vi "Construct MCListbox Item Names Binding.vi"(9 "Set to top left upon write? (F)":T1, 10 "MCListbox Refnum":refnum<vi>) -> (0 "error out":errorcluster, 3 "MCListboxItemNamesBinding":refnum<class "MCListboxItemNamesBinding.lvclass">)   [LabVIEW 2017, in "MCListboxItemNamesBinding.lvclass"]
doc: "<License>\nCopyright © 2017 Composed Systems, LLC | All rights reserved\nwww.composed.io\n\nAuthor: Ethan Stern <ethan.stern@composed.io>\n\nThis software is provided \"AS IS\" WITHOUT WARRANTIES, either express or implied, AND IS FOR EDUCATIONAL PURPOSES ONLY.\n</License>"
uses:
  MCListboxItemNamesBinding.lvclass
  MCListbox Binding Options.ctl
  MCListboxItemNamesBinding.lvclass/MCListboxItemNamesBinding.ctl
  <vilib>/Utility/error.llb/Error Cluster From Error Code.vi
  <vilib>/ErrorRing/Error Ring.xnode
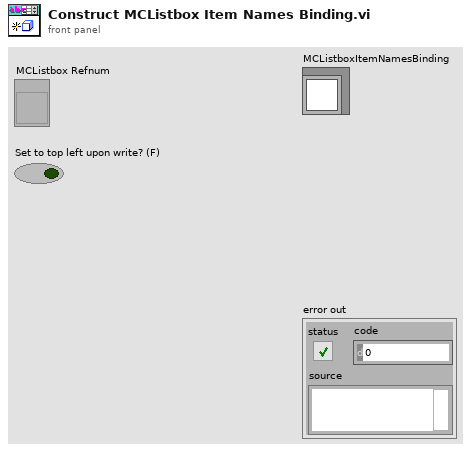
[diagram p1: front panel]
types:
  T1 = typedef "MCListboxItemNamesBinding.lvclass/MCListbox Binding Options.ctl" = bool
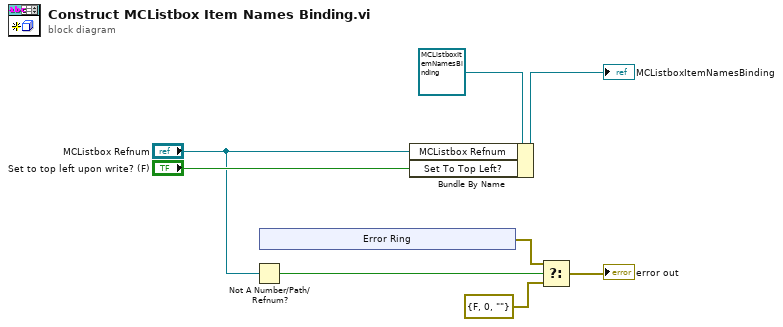
[diagram p0: block diagram]
diagram:
  n1 = Not A Number/Path/Refnum?(number/path/refnum="MCListbox Refnum") -> (NaN/Path/Refnum?=w5:bool)
  n2 = xnode "Error Ring"() -> ("error out"=w3:errorcluster)
  n3 = Bundle By Name(cluster=refnum<class "MCListboxItemNamesBinding.lvclass"> refnum ("MCListboxItemNamesBinding"), "MCListbox Refnum"="MCListbox Refnum", "Set To Top Left?"="Set to top left upon write? (F)") -> (→"MCListboxItemNamesBinding":refnum<class "MCListboxItemNamesBinding.lvclass">)
  n4 = Select(t=w3, s=w5, f=errorcluster {"status"=FALSE, "code"=0, "source"=""} ("error constant")) -> (s? t:f=→"error out":errorcluster)
